vi "Main.vi"() -> ()   [LabVIEW 2013]
uses:
  <vilib>/myRIO/Instrument Drivers/Onboard IO/I2C/typedefs/I2C User Configuration.ctl
  <vilib>/myRIO/Instrument Drivers/Onboard IO/I2C/typedefs/I2C Transfer Rate.ctl
  <vilib>/Platform/TimedLoop/XDataNode/timing_clust.ctl
  <vilib>/Platform/TimedLoop/XDataNode/nitl_modes.ctl
  <vilib>/Platform/TimedLoop/XDataNode/wakeup.ctl
  <vilib>/myRIO/Common/Instrument Driver Framework/myRIO v1.0/DIO/vis/myRIO v1.1 Open DIO.vi
  <vilib>/myRIO/Common/Instrument Driver Framework/myRIO v1.0/I2C/vis/myRIO v1.1 Open I2C.vi
  <vilib>/myRIO/Common/Instrument Driver Framework/myRIO v1.0/UART/vis/myRIO v1.0 Close UART.vi
  <vilib>/myRIO/Common/Instrument Driver Framework/Utilities/vis/Validate Channels.vi
  <vilib>/myRIO/Common/Instrument Driver Framework/myRIO v1.0/DIO/vis/myRIO v1.0 Reserve DIO.vi
  <vilib>/myRIO/Common/Instrument Driver Framework/myRIO v1.0/I2C/vis/myRIO v1.0 Reserve I2C.vi
  <vilib>/myRIO/Common/Instrument Driver Framework/myRIO v1.0/Resource Manager/vis/myRIO v1.0 Reserve Channel List.vi
  <vilib>/myRIO/Common/Instrument Driver Framework/myRIO v1.0/DIO/vis/myRIO v1.0 Build MUX Configuration DIO.vi
  <vilib>/myRIO/Common/Instrument Driver Framework/myRIO v1.0/I2C/vis/myRIO v1.0 Build MUX Configuration I2C.vi
  <vilib>/myRIO/Common/Instrument Driver Framework/myRIO v1.0/Resource Manager/vis/myRIO v1.0 Reserve Channel.vi
  <vilib>/myRIO/Common/Instrument Driver Framework/myRIO v1.0/Resource Manager/vis/myRIO v1.0 Unreserve Channel.vi
  <vilib>/myRIO/Common/Instrument Driver Framework/myRIO v1.0/Resource Manager/vis/myRIO v1.0 Create Configuration List.vi
  <vilib>/myRIO/Common/Instrument Driver Framework/myRIO v1.0/Resource Manager/vis/myRIO v1.0 Build Mutex Name.vi
  <vilib>/myRIO/Common/Instrument Driver Framework/myRIO v1.0/myRIO v1.1 Open.vi
  <vilib>/Utility/VariantDataType/GetNumericInfo.vi
  <vilib>/Utility/error.llb/Error Cluster From Error Code.vi
  <vilib>/myRIO/Common/Instrument Driver Framework/Utilities/vis/IO Manager.vi
  <vilib>/myRIO/Common/Instrument Driver Framework/Utilities/vis/Configuration Manager.vi
  <vilib>/myRIO/Common/Instrument Driver Framework/myRIO v1.0/Resource Manager/vis/myRIO v1.0 Configure IO.vi
  <vilib>/myRIO/Common/Instrument Driver Framework/myRIO v1.0/myRIO v1.0 Close.vi
  <vilib>/myRIO/Common/Instrument Driver Framework/myRIO v1.0/I2C/vis/myRIO v1.0 Configure I2C.vi
  <vilib>/myRIO/Common/Instrument Driver Framework/myRIO v1.0/I2C/vis/myRIO v1.0 Write I2C.vi
  <vilib>/myRIO/Common/Instrument Driver Framework/myRIO v1.0/DIO/vis/myRIO v1.0 Read DIO.vi
  <vilib>/myRIO/Common/Instrument Driver Framework/myRIO v1.0/I2C/vis/myRIO v1.0 Read I2C.vi
  <vilib>/myRIO/Common/Instrument Driver Framework/Utilities/vis/FPGA Ref Manager.vi
  <vilib>/myRIO/Common/Instrument Driver Framework/myRIO v1.0/myRIO v1.0 Reset FPGA.vi
  <vilib>/platform/TimedLoop/XDataNode/XDataNode.xnode
  <vilib>/myRIO/Instrument Drivers/Utilities/Utilities.lvlib
  <vilib>/Platform/TimedLoop/XDataNode/XDNodeRunTimeDep.lvlib
  <vilib>/myRIO/Instrument Drivers/Onboard IO/I2C/I2C.lvlib
  <vilib>/myRIO/Instrument Drivers/Onboard IO/DIO/DIO.lvlib
panel:
  in  "[ESC]":bool
  out "Magnetic field [LSb]":cluster{i16, i16, i16}(graph) caption="Waveform Chart"
  out "Z":i16
  out "Y":i16
  out "X":i16
  out "DATA":u8[](array[numeric]) format="%02x"
  # "Compass demo"
  # "DATA_X_H"
  # "DATA_X_L"
  # "DATA_Z_H"
  # "DATA_Z_L"
  # "DATA_Y_H"
  # "DATA_Y_L"
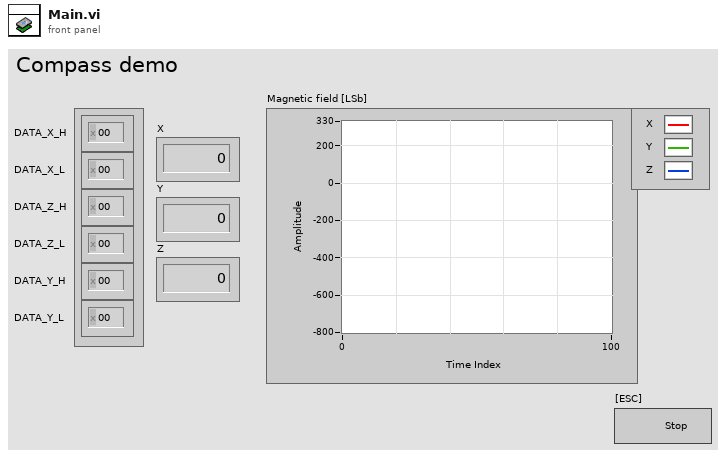
[diagram p1: front panel]
types:
  T1 = typedef "I2C.lvlib/I2C User Configuration.ctl" = cluster{"I2C Transfer Rate":T2}
  T2 = typedef "I2C.lvlib/I2C Transfer Rate.ctl" = enum16{"Standard Mode (100 kbps)", "Fast Mode (400 kbps)"}
  T3 = typedef "I2C.lvlib/I2C Reference.ctl" = cluster{"myRIO Reference":T4, "I2C Channels Enum":T8, "I2C Configuration":T9}
  T4 = typedef "myRIO Generic Hardware Reference.ctl" = cluster{"myRIO Model":T5, "myRIO Hardware Reference":T6}
  T5 = typedef "Hardware Version Enum.ctl" = enum16{"Unknown", "myRIO-1900", "myRIO-1950"}
  T6 = typedef "myRIO v1.0 Reference.ctl" = cluster{"Generic FPGA Reference":T7, "Allow multiple opens":bool}
  T7 = typedef "Generic FPGA Reference.ctl" = refnum<k20>
  T8 = typedef "I2C Channels Enum.ctl" = enum16{"Not Connected", "A/I2C", "B/I2C"}
  T9 = typedef "I2C.lvlib/I2C Configuration.ctl" = cluster{"I2C Transfer Rate":T2}
  T10 = typedef "DIO.lvlib/DIO Reference.ctl" = cluster{"myRIO Reference":T4, "DIO Channels List":T11}
  T11 = typedef "DIO Channels List.ctl" = T12[]
  T12 = typedef "DIO Channels Enum.ctl" = enum16{"Not Connected", "C/DIO0", "C/DIO1", "C/DIO2", "C/DIO3", "C/DIO4", "C/DIO5", "C/DIO6", "C/DIO7", "A/DIO0", "A/DIO1", "A/DIO2", "A/DIO3", "A/DIO4", "A/DIO5", "A/DIO6", "A/DIO7", "A/DIO8", "A/DIO9", "A/DIO10", "A/DIO11", "A/DIO12", "A/DIO13", "A/DIO14", "A/DIO15", "B/DIO0", "B/DIO1", "B/DIO2", "B/DIO3", "B/DIO4", "B/DIO5", "B/DIO6", "B/DIO7", "B/DIO8", "B/DIO9", "B/DIO10", "B/DIO11", "B/DIO12", "B/DIO13", "B/DIO14", "B/DIO15", "LED0", "LED1", "LED2", "LED3", "Button0"}
  T13 = typedef "XDNodeRunTimeDep.lvlib/timing_clust.ctl" = cluster{"Expected End [f-1]":u64, "Actual End [f-1]":u64, "Finished Late? [f-1]":bool, "Expected End [i-1]":u64, "Actual End [i-1]":u64, "Finished Late? [i-1]":bool, "Expected Start [i]":u64, "Actual Start [i]":u64, "Expected Start [f]":u64, "Actual Start [f]":u64, "Source Name":string, "Structure Name":string, "Period":i64, "Deadline":i64, "Offset":i64, "Start":i64, "Priority":i32, "Timeout":i32, "Mode":T14, "Wakeup Reason":T15, "Error":errorcluster, "Source Type":string, "Secondary Source Type":string, "Global End Time":u64, "Global Start Time":u64, "Frame Duration":u64, "Iteration Duration":u64, "Assigned CPU":i32, "I/O Scan Engine Mode":u32}
  T14 = typedef "XDNodeRunTimeDep.lvlib/nitl_modes.ctl" = enum32{"No Change", "Process missed periods, maintain original phase", "Discard missed periods, maintain original phase", "Process missed periods, ignore original phase", "Discard missed periods, ignore original phase"}
  T15 = typedef "XDNodeRunTimeDep.lvlib/wakeup.ctl" = enum32{"Normal", "Aborted", "Asynchronous wakeup", "Timing source error", "Timed loop error", "Timeout"}
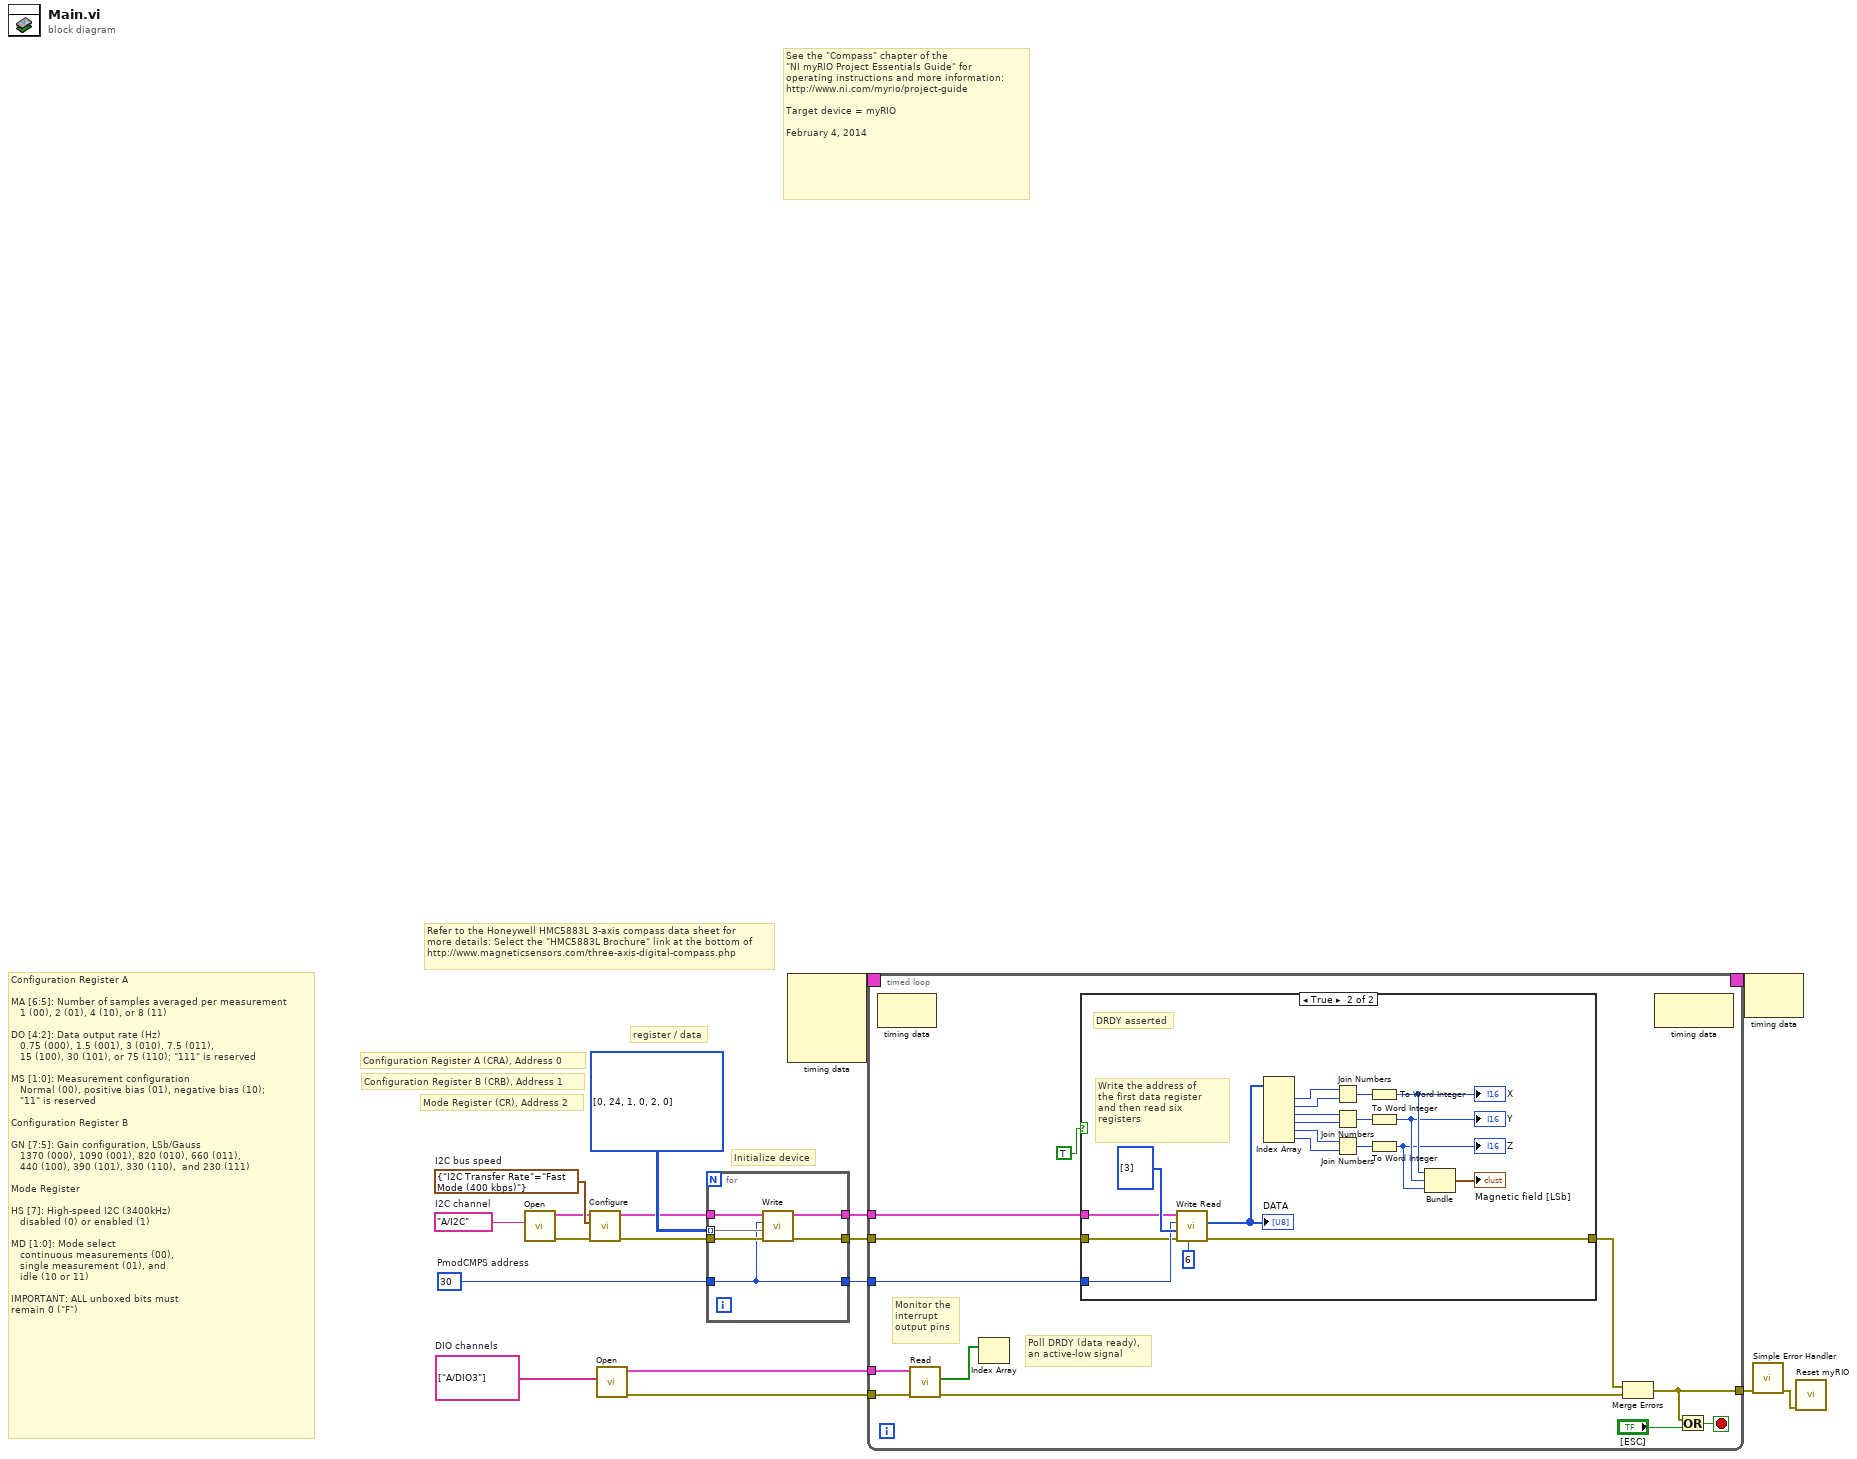
[diagram p0: block diagram]
diagram:
  w1 = tag[] ["A/DIO3"]  # DIO channels
  w13 = T1 {"I2C Transfer Rate"=enum."Fast Mode (400 kbps)"}  # I2C bus speed
  w14 = tag "A/I2C"  # I2C channel
  w4 = u8 30  # PmodCMPS address
  # "Initialize device"
  # "register / data"
  # "See the \"Compass\" chapter of the\n\"NI myRIO Project Essentials Guide\" for\noperating instructions and more information: \nhttp://www.ni.com/myrio/project-guide\n\nTarget device = myRIO\n\nFebruary 4, 2014"
  # "Refer to the Honeywell HMC5883L 3-axis compass data sheet for \nmore details: Select the \"HMC5883L Brochure\" link at the bottom of\nhttp://www.magneticsensors.com/three-axis-digital-compass.php"
  # "Configuration Register A\n\nMA [6:5]: Number of samples averaged per measurement\n   1 (00), 2 (01), 4 (10), or 8 (11)\n\nDO [4:2]: Data output rate (Hz)\n   0.75 (000), 1.5 (001), 3 (010), 7.5 (011),\n   15 (100), 30 (101), or 75 (110); \"111\" is reserved\n\nMS [1:0]: Measurement configuration\n   Normal (00), positive bias (01), negative bias (10);\n   \"11\" is reserved\n\nConfiguration Register B\n\nGN [7:5]: Gain configuration, LSb/Gauss\n   1370 (000), 1090 (001), 820 (010), 660 (011),\n   440 (100), 390 (101), 330 (110),  and 230 (111)\n\nMode Register\n\nHS [7]: High-speed I2C (3400kHz)\n   disabled (0) or enabled (1)\n\nMD [1:0]: Mode select\n   continuous measurements (00),\n   single measurement (01), and\n   idle (10 or 11)\n\nIMPORTANT: ALL unboxed bits must\nremain 0 (\"F\")"
  # "Mode Register (CR), Address 2"
  # "Configuration Register B (CRB), Address 1"
  # "Configuration Register A (CRA), Address 0"
  n1 = call <vilib>:"Open.vi"("Channel Name"=w14) -> ("error out"=w11:errorcluster, "I2C Ref Out"=w12:T3)  [unwired: 9 in]
  n2 = call <vilib>:"Configure.vi"("error in (no error)"=w11, "I2C User Configuration"=w13, "I2C Ref In"=w12) -> ("error out"=w5:errorcluster, "I2C Ref Out"=w6:T3)  [unwired: 7 in]
  n3 = call <vilib>:"Open.vi"("Channel Names"=w1) -> ("error out"=w3:errorcluster, "DIO Ref Out"=w2:T10)  [unwired: 9 in]
  n4 = for {
    tunnel: [w24] -> w10
    tunnel: [w23] -> w9
    tunnel: [w19] -> w8
    tunnel: u8[][] [[0, 24], [1, 0], [2, 0]] ("Bytes to Write") -> [w22] mode=indexing
    tunnel: w6 -> [w21]
    tunnel: w5 -> [w20]
    tunnel: w4 -> [w19]
    n5 = call <vilib>:"Write.vi"("error in (no error)"=w20, "Bytes to Write"=w22, "Slave Address (7-bit)"=w19, "I2C Ref In"=w21) -> ("error out"=w24:errorcluster, "I2C Ref Out"=w23:T3)  [unwired: 6 in]
  }
  n6 = node-c288() -> (w18:T13)  [unwired: 4 in]
  n7 = timed-loop {
    tunnel: [w27] -> w15
    tunnel: w8 -> [w32]
    tunnel: w10 -> [w34]
    tunnel: w9 -> [w33]
    tunnel: w3 -> [w31]
    tunnel: w2 -> [w30]
    timing: w18 -> [_]
    timing-out: [_] -> w17
    stop <- w36 stop-if-true
    # "Poll DRDY (data ready),\nan active-low signal"
    # "Monitor the\ninterrupt\noutput pins"
    n8 = node-c288() -> ()  [unwired: 1 in, 1 out]
    n9 = call <vilib>:"Read.vi"("error in (no error)"=w31, "DIO Ref In"=w30) -> ("error out"=w26:errorcluster, "Values"=w28:bool[])  [unwired: 7 in, 1 out]
    n10 = Index Array(array=w28) -> ()  [unwired: 1 in, 1 out]
    n11 = case shown="True" TRUE {
      tunnel: w34 -> [w39 w51]
      tunnel: w33 -> [_ w52]
      tunnel: w32 -> [_ w54]
      tunnel: [w39 w53] -> w29
      frame False {
        # "DRDY deasserted"
      }
      frame True {
        # "DRDY asserted"
        # "Write the address of\nthe first data register\nand then read six registers"
        n12 = call <vilib>:"Write Read.vi"("Byte Count"=u32 6, "error in (no error)"=w51, "Bytes to Write"=u8[] [3], "Slave Address (7-bit)"=w54, "I2C Ref In"=w52) -> ("error out"=w53:errorcluster, "Bytes Read"=w50:u8[])  [unwired: 3 in, 1 out]
        "DATA" <- w50
        n13 = Index Array(array=w50) -> (element #1=w45:u8, element #2=w44:u8, element #3=w43:u8, element #4=w42:u8, element #5=w41:u8, element #6=w40:u8)  [unwired: 6 in]
        n14 = Join Numbers(hi=w45, lo=w44) -> ((hi.lo)=w59:u16)
        n15 = Join Numbers(hi=w43, lo=w42) -> ((hi.lo)=w58:u16)
        n16 = Join Numbers(hi=w41, lo=w40) -> ((hi.lo)=w57:u16)
        n17 = To Word Integer(number=w59) -> (16bit integer=w49:i16)
        "X" <- w49
        n18 = To Word Integer(number=w58) -> (16bit integer=w48:i16)
        "Y" <- w48
        n19 = To Word Integer(number=w57) -> (16bit integer=w47:i16)
        "Z" <- w47
        n20 = Bundle(w49, w48, w47) -> (→"Magnetic field [LSb]":cluster{i16, i16, i16})  [unwired: 1 in]
      }
    }
    n21 = Merge Errors "Merge Errors"(w29, w26) -> (w27:errorcluster)
    n22 = node-c288() -> ()  [unwired: 1 in, 1 out]
    n23 = Or(x=w27, y="[ESC]") -> (x .or. y?=w36:bool)
  }
  n24 = node-c288(w17) -> ()  [unwired: 1 out]
  n25 = call <vilib>:"Simple Error Handler.vi"("error in (no error)"=w15) -> ("error out"=w16:errorcluster)  [unwired: 4 in, 4 out]
  n26 = call <vilib>:"Reset myRIO.vi"("error in (no error)"=w16) -> ()  [unwired: 10 in, 1 out]
